vi "Message to All Monkeys in the Process.vi"(0 "Tamer in":refnum<class "Tamer.lvclass">, 5 "Process ID":string, 7 "Message":string, 9 "Data":variant, 11 "error in (no error)":errorcluster) -> (4 "Tamer out":refnum<class "Tamer.lvclass">, 15 "error out":errorcluster)   [LabVIEW 2020, in "TALOS.lvlib" / "Tamer.lvlib" / "Tamer.lvclass"]
uses:
  Tamer.lvclass
  C:/LabVIEW Code/TALOS/talos/Father of all uServices/Father of all uServices/Father of all uServices.lvclass
  Guardian/Guardian Messages/Message to uService Msg/Message to uService Msg.lvclass/Message to uService Msg.ctl
  Ancestor/Ancestor/Ancestor.lvclass/Ancestor.ctl
  Guardian/Guardian Messages/Message to uService Msg/Send Message to uService.vi
  Support VIs/Substitute Error.vi
  FGV/Error Memory/Get Error Description.vi
  Support VIs/Get PC name.vi
  Ancestor/Ancestor/Read ID.vi
  Support VIs/Get Class Name.vi
  <vilib>/Utility/error.llb/Clear Errors.vi
  FGV/Error Memory/Error Memory Core.vi
  <vilib>/AdvancedString/Delimited String to 1D String Array.vi
  Support VIs/Circus Root Path.vi
  FGV/Error Memory/Error Crt Lvl checker.vi
  FGV/Error Memory/Error Memory Core.vi/40c8088d-b597-4017-91af-faa98e00292e.vi
  FGV/Error Memory/Error Memory Core.vi/d4a3ab98-063c-4e44-b43d-fbdcfe6c2be2.vi
  Father of all uServices/Father of all uServices/Father of all uServices.lvclass
  C:/LabVIEW Code/TALOS/builds/Actor Framework PPL/Actor Framework.lvlibp/1abvi3w/vi.lib/ActorFramework/Actor/Actor.lvclass
  builds/Actor Framework PPL/Actor Framework.lvlibp/1abvi3w/vi.lib/ActorFramework/Actor/Read Caller Enqueuer.vi
  builds/Actor Framework PPL/Actor Framework.lvlibp/1abvi3w/vi.lib/ActorFramework/Message Enqueuer/Enqueue.vi
  Support VIs/Global Memory.vi
  <vilib>/Utility/LVClass/Get LV Class Name.vi
  Support VIs/Is in Packed Library.vi
  Support VIs/TALOS Root path.vi
  Support VIs/Read CSV worksheet.vi
  Support VIs/Global Constants.vi
  <vilib>/Utility/error.llb/General Error Handler.vi
  Support VIs/Error Log.vi
  Guardian/Guardian Messages/Message to uService Msg/Message to uService Msg.lvclass
  Ancestor/Ancestor/Ancestor.lvclass
  <vilib>/Comparison/Equal/Equal Functor/Equal Functor.lvclass
  TALOS.lvlib
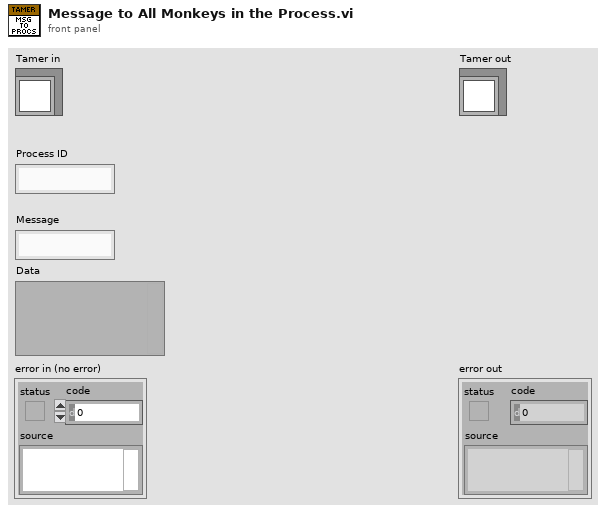
[diagram p1: front panel]
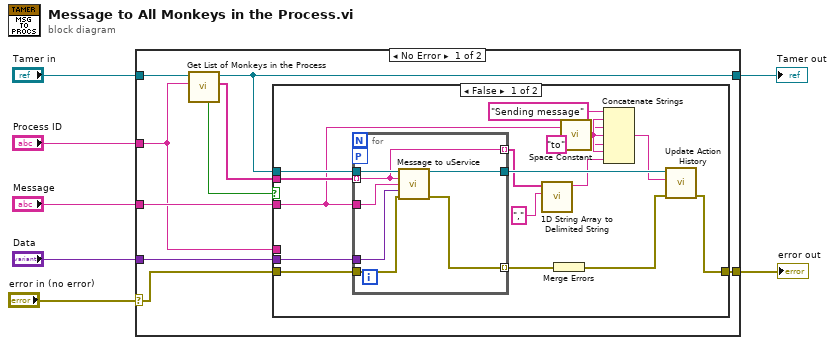
[diagram p0: block diagram]
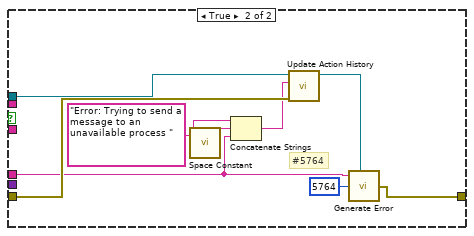
[diagram p2: hidden frame]
diagram:
  n1 = case shown="No Error" "error in (no error)" {
    selector: "error in (no error)" -> [w13 w50]
    tunnel: [w14 w50] -> w6
    tunnel: [w11 w49] -> w4
    tunnel: "Tamer in" -> [w12 w49]
    tunnel: "Message" -> [w16 _]
    tunnel: "Data" -> [w15 _]
    tunnel: "Process ID" -> [w10 _]
    frame No Error {
      n2 = call-dynamic "Get List of Monkeys in the Process.vi"("Process ID"=w10, "Tamer in"=w12) -> ("List of Monkeys"=w9:string[], "Tamer out"=w11:refnum<class "Tamer.lvclass">, "Process not found?"=w8:bool)  [unwired: 6 in, 1 out]
      n3 = case shown="False" w8 {
        tunnel: w16 -> [w19 _]
        tunnel: w15 -> [w32 _]
        tunnel: [w28 w48] -> w14
        tunnel: w13 -> [w31 w44]
        tunnel: w9 -> [w30 _]
        tunnel: w11 -> [w29 w46]
        tunnel: w10 -> [_ w41]
        frame False {
          n4 = for {
            tunnel: w19 -> [w37]
            tunnel: w32 -> [w39]
            tunnel: w30 -> [w35] mode=indexing
            tunnel: [w35] -> w23 mode=indexing
            tunnel: w31 -> [w34]
            tunnel: [w33] -> w18 mode=indexing
            tunnel: w29 -> [w38]
            tunnel: [w36] -> w27
            workers-P: _ -> [_]
            n5 = call "Message to uService.vi"("Father of all uServices in"=w38, "uService ID"=w35, "Message"=w37, "Data"=w39, "error in (no error)"=w34) -> ("Father of all uServices out"=w36:refnum<class "Tamer.lvclass">, "error out"=w33:errorcluster)  [unwired: 9 in]
          }
          n6 = call <vilib>:"1D String Array to Delimited String.vi"("delimiter"="," ("Separator"), "string array"=w23) -> ("delimited string"=w21:string)  [unwired: 9 in]
          n7 = Merge Errors(w18) -> (w17:errorcluster)
          n8 = call <vilib>:"Space Constant.vi"() -> ("String"=w26:string)
          n9 = Concatenate Strings("Sending message" ("string"), w26, w19, w26, "to" ("string"), w26, w21) -> (w20:string)
          n10 = call-dynamic "Update Action History.vi"("error in (no error)"=w17, "Action"=w20, "Tamer in"=w27) -> ("error out"=w28:errorcluster)  [unwired: 7 in, 1 out]
        }
        frame True {
          # "#5764"
          n11 = call <vilib>:"Space Constant.vi"() -> ("String"=w40:string)
          n12 = Concatenate Strings("Error: Trying to send a message to an unavailable process " ("Action"), w40, w41) -> (w42:string)
          n13 = call-dynamic "Update Action History.vi"("error in (no error)"=w44, "Action"=w42, "Tamer in"=w46) -> ("Tamer out"=w45:refnum<class "Tamer.lvclass">)  [unwired: 7 in, 1 out]
          n14 = call "Generate Error.vi"("Optional String"=w41, "Class"=w45, "Error Code"=5764) -> ("error out"=w48:errorcluster)  [unwired: 4 in]
        }
      }
    }
    frame Error {
    }
  }
  "error out" <- w6
  "Tamer out" <- w4
